vi "Pressure_History.vi"() -> ()   [LabVIEW 2015]
panel:
  out "XY Graph":cluster{cluster{"Comment":timestamp, dbl}[]}[](graph)
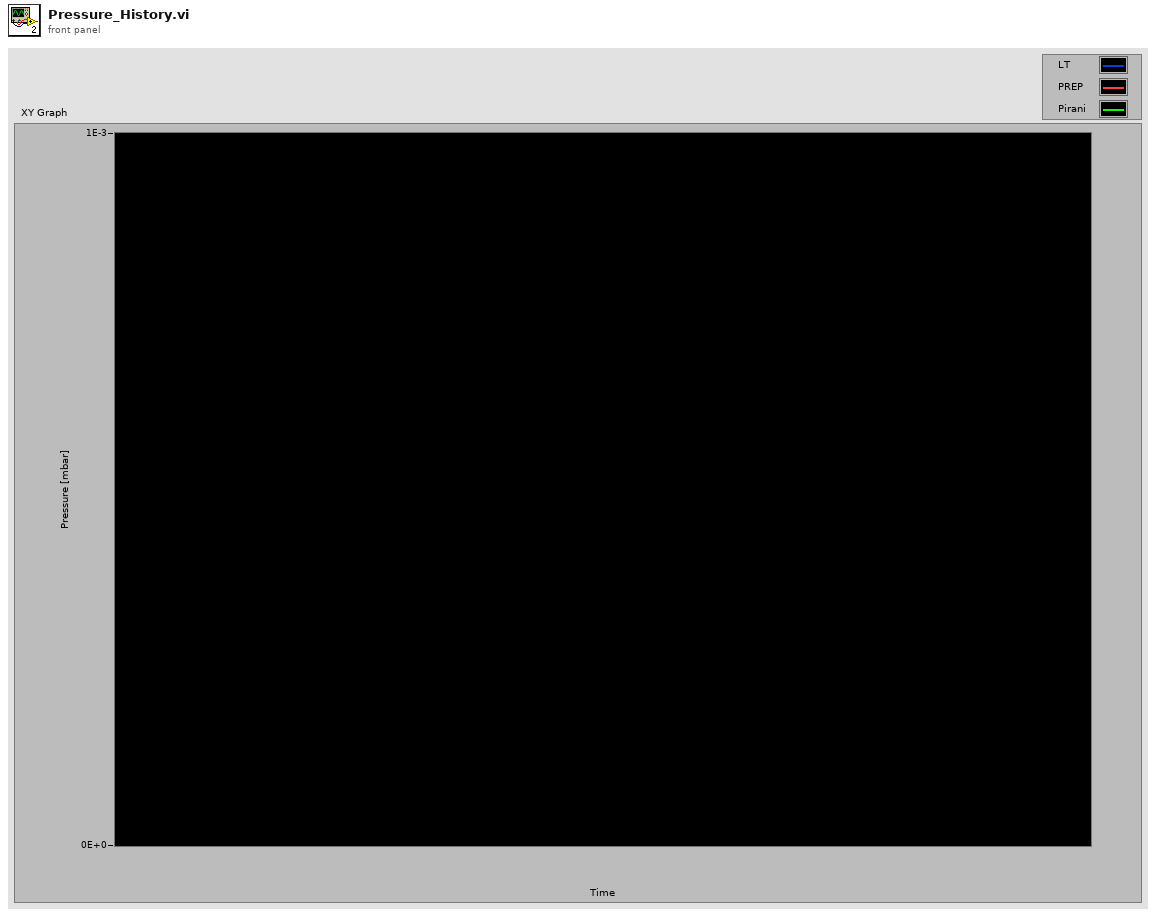
[diagram p1: front panel]
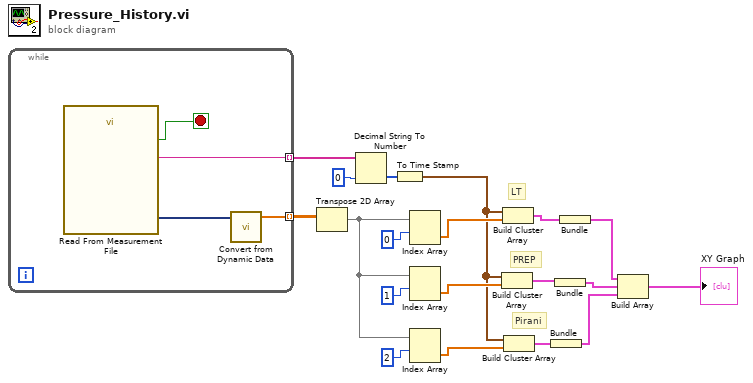
[diagram p0: block diagram]
diagram:
  # "Pirani"
  # "PREP"
  # "LT"
  n1 = while {
    tunnel: [w21] -> w16 mode=indexing
    tunnel: [w20] -> w19 mode=indexing
    stop <- w23 stop-if-true
    n2 = call "Read From Measurement File"() -> ("Signals"=w22:dynamicdata, "EOF?"=w23:bool, "Comment"=w20:string)  [unwired: 6 in, 3 out]
    n3 = call "Convert from Dynamic Data"("Dynamic Data Type"=w22) -> ("Array"=w21:dbl[])  [unwired: 3 in]
  }
  n4 = Transpose 2D Array(2D array=w16) -> (transposed array=w12:dbl[][])
  n5 = Decimal String To Number(string=w19, default (0L)=i64 0 ("default (0 I32)")) -> (number=w15:i64[])  [unwired: 1 in, 1 out]
  n6 = To Time Stamp(1:w15) -> (0:w8:timestamp[])
  n7 = Index Array(array=w12, index (row)=0) -> (element=w11:dbl[])  [unwired: 1 in]
  n8 = Index Array(array=w12, index (row)=1) -> (element=w10:dbl[])  [unwired: 1 in]
  n9 = Index Array(array=w12, index (row)=2) -> (element=w9:dbl[])  [unwired: 1 in]
  n10 = Build Cluster Array(w8, w10) -> (w6:cluster{"Comment":timestamp, dbl}[])
  n11 = Build Cluster Array(w8, w11) -> (w7:cluster{"Comment":timestamp, dbl}[])
  n12 = Build Cluster Array(w8, w9) -> (w5:cluster{"Comment":timestamp, dbl}[])
  n13 = Bundle(w5) -> (w2:cluster{cluster{"Comment":timestamp, dbl}[]})  [unwired: 1 in]
  n14 = Bundle(w6) -> (w3:cluster{cluster{"Comment":timestamp, dbl}[]})  [unwired: 1 in]
  n15 = Bundle(w7) -> (w4:cluster{cluster{"Comment":timestamp, dbl}[]})  [unwired: 1 in]
  n16 = Build Array(w4, w3, w2) -> (→"XY Graph":cluster{cluster{"Comment":timestamp, dbl}[]}[])
